vi "TriggerDialog.vi"(8 "Error In":errorcluster, 11 "Trigger Configuration In":T2={"Input"={"Type"=enum."None", "Timeout (ms)"=0, "Delay (ms)"=0, "Digital IO Line (1-14)"=0, "Digital IO Mode"=enum."Falling"}, "Output"={"Type"=enum."None", "Delay (ms)"=0, "Digital IO Line (1-14)"=1, "Digital IO Mode"=enum."Falling", "Digital IO Pulse Width (sec)"=0.0}} {"Output"."Digital IO Line (1-14)" min=1 max=14 step=1}) -> (0 "Error Out":errorcluster, 2 "Cancelled":bool, 3 "Trigger Configuration Out":T2={"Input"={"Type"=enum."None", "Timeout (ms)"=0, "Delay (ms)"=0, "Digital IO Line (1-14)"=0, "Digital IO Mode"=enum."Falling"}, "Output"={"Type"=enum."None", "Delay (ms)"=0, "Digital IO Line (1-14)"=1, "Digital IO Mode"=enum."Falling", "Digital IO Pulse Width (sec)"=0.0}} {"Output"."Digital IO Line (1-14)" min=1 max=14 step=1})   [LabVIEW 2013]
uses:
  TriggerConfiguration.ctl
  TriggerInputConfiguration.ctl
  TriggerInputType.ctl
  driver/Public/Controls/TriggerMode.ctl
  TriggerOutputConfiguration.ctl
  TriggerOutputType.ctl
  driver/Keithley-2602.lvlib
  libs/LV-Utilities/LV-Utilities.lvlib
panel:
  in  "Input Timeout (msec)":u32
  in  "Input Delay (msec)":u32
  in  "Input Mode":T1(ring)
  in  "Input Digital IO Channel":u8=1 min=1 max=14 step=1
  in  "Input Type":enum16{"None", "Digital IO", "Bus"}(ring)
  in  "Output Delay (msec)":u32
  in  "Output Pulse Width (sec)":dbl format="%_4p"
  in  "Output Mode":T1(ring)
  in  "Output Digital IO Channel":u8=1 min=1 max=14 step=1
  in  "Output Type":enum16{"None", "Digital IO", "Bus"}(ring)
  in  "CANCEL":bool
  in  "DONE":bool
  # "INPUT"
  # "Timeout"
  # "Delay"
  # "Mode"
  # "Line"
  # "Type"
  # "OUTPUT"
  # "Delay"
  # "Pulse Width"
  # "Mode"
  # "Line"
  # "Type"
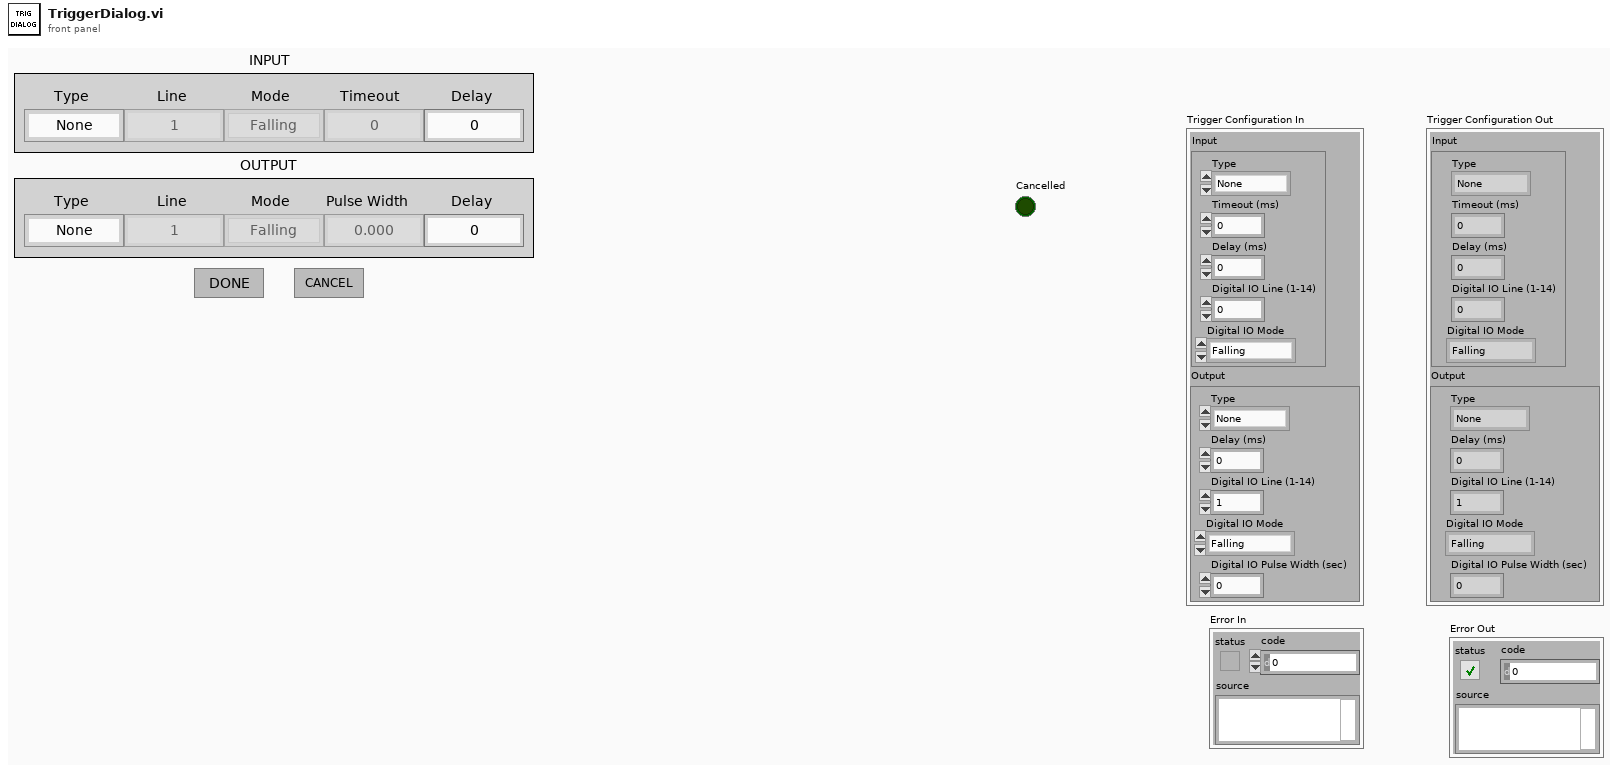
[diagram p1: front panel]
types:
  T1 = enum16{"Falling", "Rising", "Either", "Synchronous"}
  T2 = typedef "TriggerConfiguration.ctl" = cluster{"Input":T3, "Output":T6}
  T3 = typedef "TriggerInputConfiguration.ctl" = cluster{"Type":T4, "Timeout (ms)":u32, "Delay (ms)":u32, "Digital IO Line (1-14)":u8, "Digital IO Mode":T5}
  T4 = typedef "TriggerInputType.ctl" = enum16{"None", "Digital IO", "Bus"}
  T5 = typedef "Keithley-2602.lvlib/TriggerMode.ctl" = enum16{"Falling", "Rising", "Either", "Synchronous"}
  T6 = typedef "TriggerOutputConfiguration.ctl" = cluster{"Type":T7, "Delay (ms)":u32, "Digital IO Line (1-14)":u8, "Digital IO Mode":T5, "Digital IO Pulse Width (sec)":dbl}
  T7 = typedef "TriggerOutputType.ctl" = enum16{"None", "Digital IO", "Bus"}
  T8 = enum8{"Enabled", "Disabled", "Disabled and Grayed Out"}
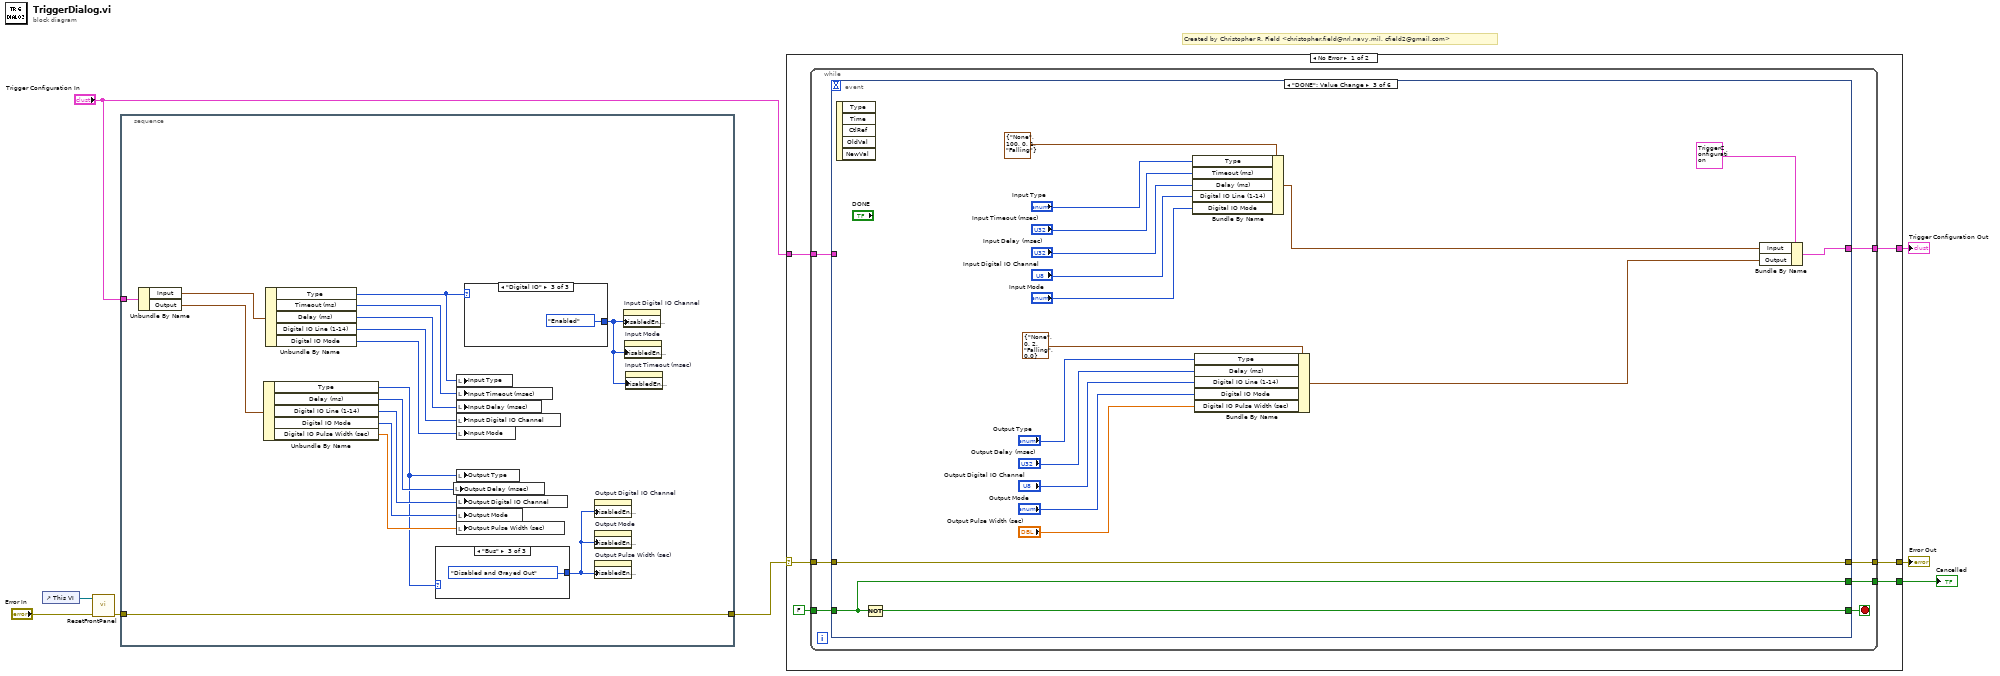
[diagram p0: block diagram]
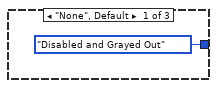
[diagram p2: hidden frame]
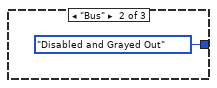
[diagram p3: hidden frame]
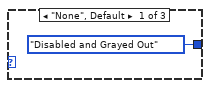
[diagram p4: hidden frame]
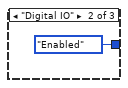
[diagram p5: hidden frame]
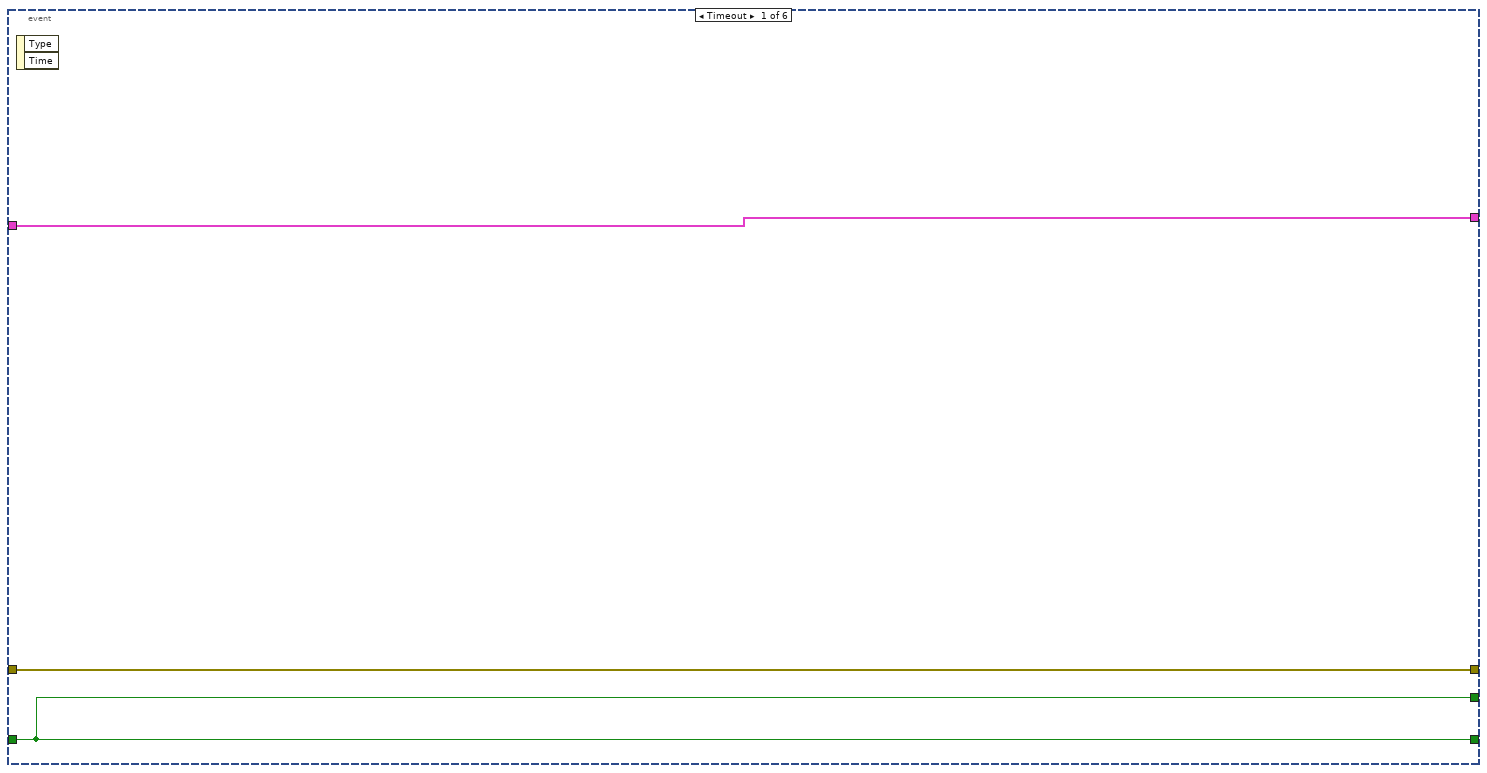
[diagram p6: hidden frame]
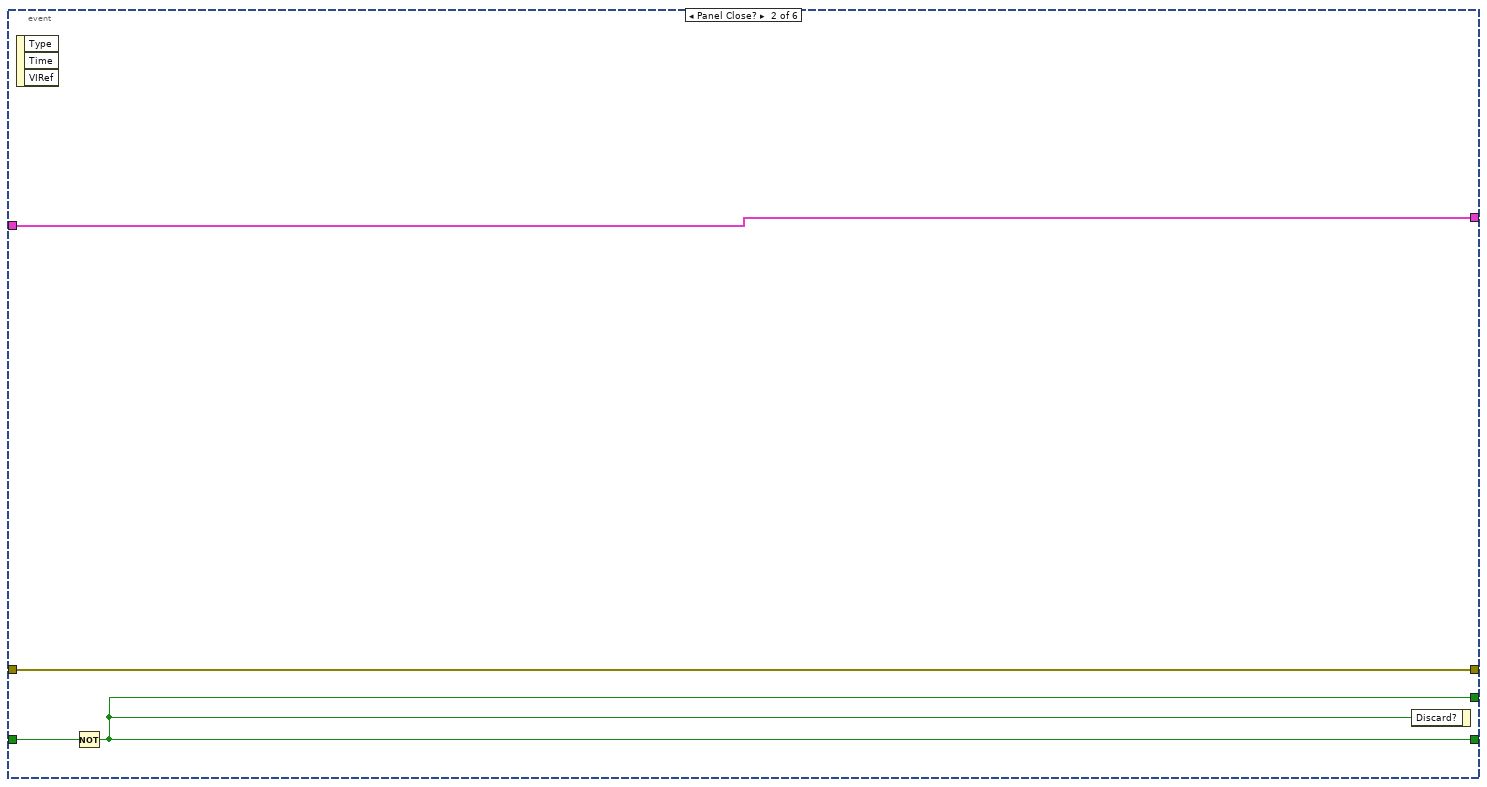
[diagram p7: hidden frame]
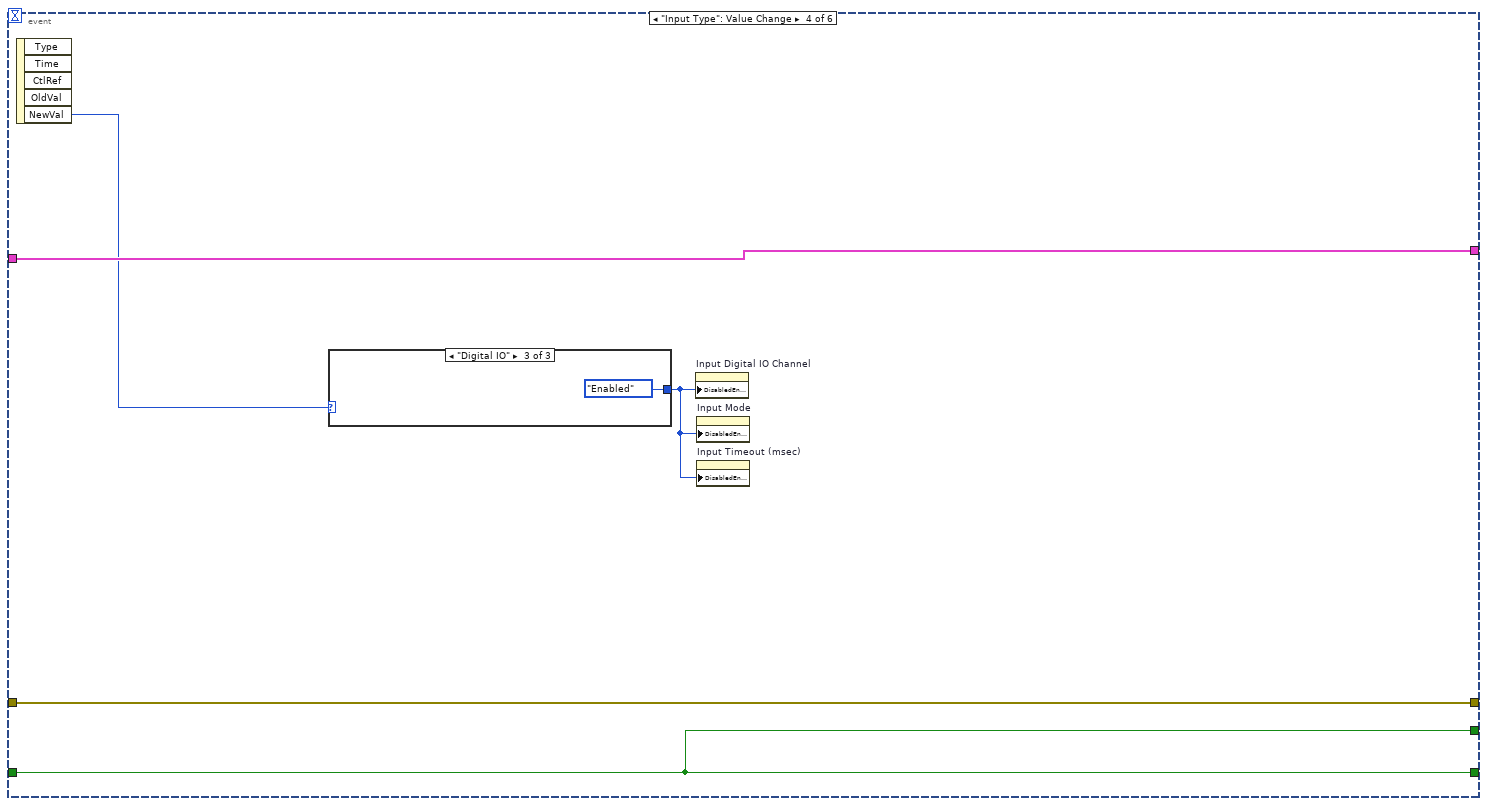
[diagram p8: hidden frame]
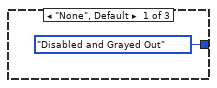
[diagram p9: hidden frame]
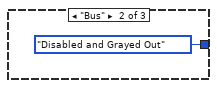
[diagram p10: hidden frame]
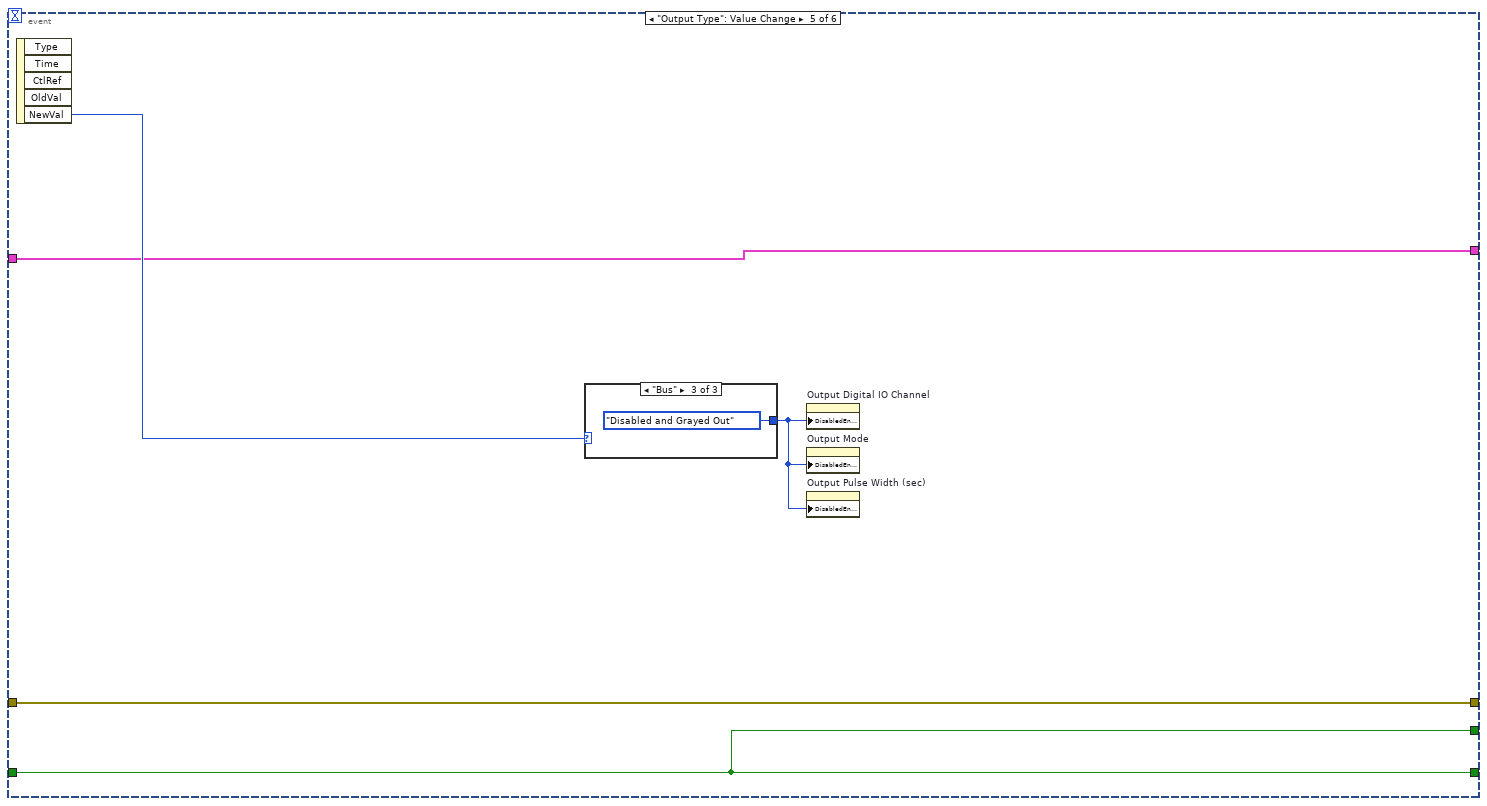
[diagram p11: hidden frame]
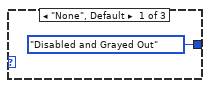
[diagram p12: hidden frame]
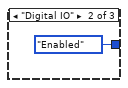
[diagram p13: hidden frame]
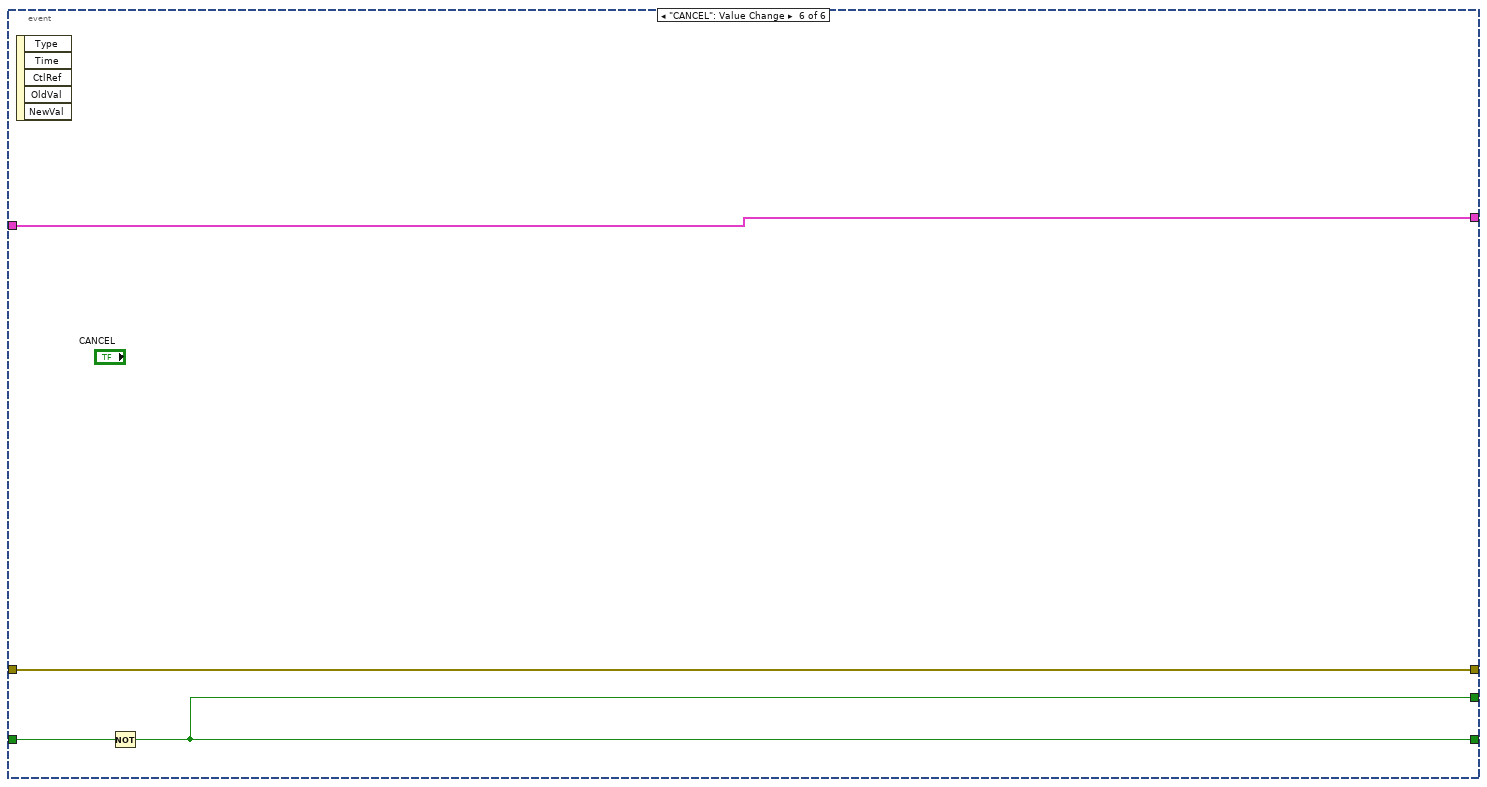
[diagram p14: hidden frame]
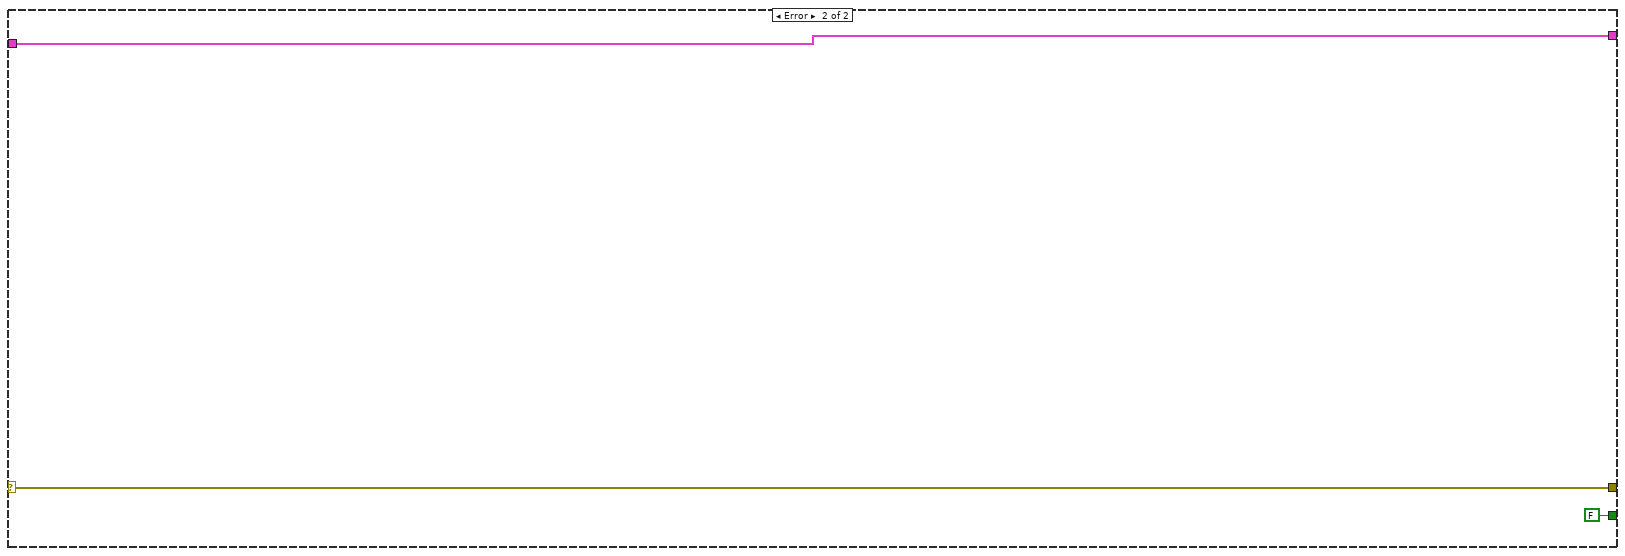
[diagram p15: hidden frame]
diagram:
  # "Created by Christopher R. Field <christopher.field@nrl.navy.mil, cfield2@gmail.com>"
  n1 = control-ref of="This VI"() -> (w1:refnum<vi>)
  n2 = call "ResetFrontPanel.vi"("Error In"="Error In", "VI Ref In"=w1) -> ("Error Out"=w5:errorcluster)  [unwired: 8 in, 1 out]
  n3 = stacked-sequence {
    tunnel: "Trigger Configuration In" -> [w23]
    tunnel: w5 -> [w24]
    tunnel: [w24] -> w4
    frame #0 {
      n4 = Unbundle By Name(w23) -> ("Input"=w22:T3, "Output"=w17:T6)
      n5 = Unbundle By Name(w17) -> ("Type"=w11:T7, "Delay (ms)"=w16:u32, "Digital IO Line (1-14)"=w15:u8, "Digital IO Mode"=w14:T5, "Digital IO Pulse Width (sec)"=w13:dbl)
      n6 = Unbundle By Name(w22) -> ("Type"=w10:T4, "Timeout (ms)"=w21:u32, "Delay (ms)"=w20:u32, "Digital IO Line (1-14)"=w19:u8, "Digital IO Mode"=w18:T5)
      n7 = case shown="\"Bus\"" w11 {
        tunnel: [T8."Disabled and Grayed Out" ("Disabled") T8."Enabled" ("Disabled") T8."Disabled and Grayed Out" ("Disabled")] -> w12
        frame "None", Default {
        }
        frame "Digital IO" {
        }
        frame "Bus" {
        }
      }
      n8 = local write "Output Delay (msec)"(w16) -> ()
      n9 = local write "Input Type"(w10) -> ()
      n10 = local write "Input Timeout (msec)"(w21) -> ()
      n11 = local write "Input Delay (msec)"(w20) -> ()
      n12 = local write "Input Digital IO Channel"(w19) -> ()
      n13 = local write "Input Mode"(w18) -> ()
      n14 = local write "Output Type"(w11) -> ()
      n15 = local write "Output Digital IO Channel"(w15) -> ()
      n16 = local write "Output Mode"(w14) -> ()
      n17 = local write "Output Pulse Width (sec)"(w13) -> ()
      n18 = case shown="\"Digital IO\"" w10 {
        tunnel: [T8."Disabled and Grayed Out" ("Disabled") T8."Disabled and Grayed Out" ("Disabled") T8."Enabled" ("Disabled")] -> w9
        frame "None", Default {
        }
        frame "Bus" {
        }
        frame "Digital IO" {
        }
      }
      n19 = property on="Output Digital IO Channel" class="DigNum (strict)"("DisabledEnum"=w12) -> ()  [unwired: 2 in, 2 out]
      n20 = property on="Output Mode" class="Enum (strict)"("DisabledEnum"=w12) -> ()  [unwired: 2 in, 2 out]
      n21 = property on="Output Pulse Width (sec)" class="DigNum (strict)"("DisabledEnum"=w12) -> ()  [unwired: 2 in, 2 out]
      n22 = property on="Input Digital IO Channel" class="DigNum (strict)"("DisabledEnum"=w9) -> ()  [unwired: 2 in, 2 out]
      n23 = property on="Input Mode" class="Enum (strict)"("DisabledEnum"=w9) -> ()  [unwired: 2 in, 2 out]
      n24 = property on="Input Timeout (msec)" class="DigNum (strict)"("DisabledEnum"=w9) -> ()  [unwired: 2 in, 2 out]
    }
  }
  n25 = case shown="No Error" w4 {
    selector: w4 -> [w32 w90]
    tunnel: [w35 FALSE] -> w8
    tunnel: [w34 w92] -> w7
    tunnel: "Trigger Configuration In" -> [w33 w92]
    tunnel: [w31 w90] -> w3
    frame No Error {
      n26 = while {
        tunnel: FALSE -> [w43]
        tunnel: [w41] -> w35
        tunnel: [w40] -> w34
        tunnel: w33 -> [w39]
        tunnel: w32 -> [w38]
        tunnel: [w37] -> w31
        stop <- w42 stop-if-true
        n27 = event shown="[2] \"DONE\": Value Change" {
          selector: _ -> [_ _ _ _ _ _]
          dyn-events: _ -> [_ _ _ _ _ _]
          timeout: _ -> [_ _ _ _ _ _]
          tunnel: w43 -> [w46 w50 w68 w72 w78 w89]
          tunnel: [w46 w49 w69 w72 w78 w88] -> w42
          tunnel: [w46 w49 w68 w72 w78 w88] -> w41
          tunnel: [w45 w48 w53 w74 w81 w87] -> w40
          tunnel: w39 -> [w45 w48 _ w74 w81 w87]
          tunnel: w38 -> [w44 w47 w52 w73 w79 w86]
          tunnel: [w44 w47 w52 w73 w79 w86] -> w37
          event Timeout {
            n28 = event-data() -> ()  [unwired: 1 in, 2 out]
          }
          event Panel Close? {
            n29 = event-data() -> ()  [unwired: 1 in, 3 out]
            n30 = Not(x=w50) -> (.not. x?=w49:bool)
            n31 = event-data("Discard?"=w49) -> ()  [unwired: 1 in, 1 out]
          }
          event "DONE": Value Change {
            n32 = event-data() -> ()  [unwired: 1 in, 5 out]
            n33 = Not(x=w68) -> (.not. x?=w69:bool)
            n34 = Bundle By Name(cluster=T3 {"Type"=enum."None", "Timeout (ms)"=100, "Delay (ms)"=0, "Digital IO Line (1-14)"=1, "Digital IO Mode"=enum."Falling"} ("Trigger Input Configuration"), "Type"="Input Type", "Timeout (ms)"="Input Timeout (msec)", "Delay (ms)"="Input Delay (msec)", "Digital IO Line (1-14)"="Input Digital IO Channel", "Digital IO Mode"="Input Mode") -> (w55:T3)
            n35 = Bundle By Name(cluster=T6 {"Type"=enum."None", "Delay (ms)"=0, "Digital IO Line (1-14)"=2, "Digital IO Mode"=enum."Falling", "Digital IO Pulse Width (sec)"=0.0} ("Output Trigger Configuration"), "Type"="Output Type", "Delay (ms)"="Output Delay (msec)", "Digital IO Line (1-14)"="Output Digital IO Channel", "Digital IO Mode"="Output Mode", "Digital IO Pulse Width (sec)"="Output Pulse Width (sec)") -> (w54:T6)
            n36 = Bundle By Name(cluster=T2 {"Input"={"Type"=enum."None", "Timeout (ms)"=0, "Delay (ms)"=0, "Digital IO Line (1-14)"=0, "Digital IO Mode"=enum."Falling"}, "Output"={"Type"=enum."None", "Delay (ms)"=0, "Digital IO Line (1-14)"=1, "Digital IO Mode"=enum."Falling", "Digital IO Pulse Width (sec)"=0.0}} ("Trigger Configuration"), "Input"=w55, "Output"=w54) -> (w53:T2)
          }
          event "Input Type": Value Change {
            n37 = event-data() -> ("NewVal"=w71:enum16{"None", "Digital IO", "Bus"})  [unwired: 1 in, 4 out]
            n38 = case shown="\"Digital IO\"" w71 {
              tunnel: [T8."Disabled and Grayed Out" ("Disabled") T8."Disabled and Grayed Out" ("Disabled") T8."Enabled" ("Disabled")] -> w70
              frame "None", Default {
              }
              frame "Bus" {
              }
              frame "Digital IO" {
              }
            }
            n39 = property on="Input Digital IO Channel" class="DigNum (strict)"("DisabledEnum"=w70) -> ()  [unwired: 2 in, 2 out]
            n40 = property on="Input Mode" class="Enum (strict)"("DisabledEnum"=w70) -> ()  [unwired: 2 in, 2 out]
            n41 = property on="Input Timeout (msec)" class="DigNum (strict)"("DisabledEnum"=w70) -> ()  [unwired: 2 in, 2 out]
          }
          event "Output Type": Value Change {
            n42 = event-data() -> ("NewVal"=w82:enum16{"None", "Digital IO", "Bus"})  [unwired: 1 in, 4 out]
            n43 = case shown="\"Bus\"" w82 {
              tunnel: [T8."Disabled and Grayed Out" ("Disabled") T8."Enabled" ("Disabled") T8."Disabled and Grayed Out" ("Disabled")] -> w80
              frame "None", Default {
              }
              frame "Digital IO" {
              }
              frame "Bus" {
              }
            }
            n44 = property on="Output Digital IO Channel" class="DigNum (strict)"("DisabledEnum"=w80) -> ()  [unwired: 2 in, 2 out]
            n45 = property on="Output Mode" class="Enum (strict)"("DisabledEnum"=w80) -> ()  [unwired: 2 in, 2 out]
            n46 = property on="Output Pulse Width (sec)" class="DigNum (strict)"("DisabledEnum"=w80) -> ()  [unwired: 2 in, 2 out]
          }
          event "CANCEL": Value Change {
            n47 = event-data() -> ()  [unwired: 1 in, 5 out]
            n48 = Not(x=w89) -> (.not. x?=w88:bool)
          }
        }
      }
    }
    frame Error {
    }
  }
  "Cancelled" <- w8
  "Trigger Configuration Out" <- w7
  "Error Out" <- w3
